vi "Random Strip Chart_v1.vi"() -> ()   [LabVIEW 2026]
panel:
  out "Numeric 3":dbl
  in  "Numeric 2":dbl
  in  "Numeric":dbl
  in  "Loop time (ms)":dbl(knob) scale=0.0..1000.0
  out "Waveform Chart":dbl(graph)
  in  "Stop":bool
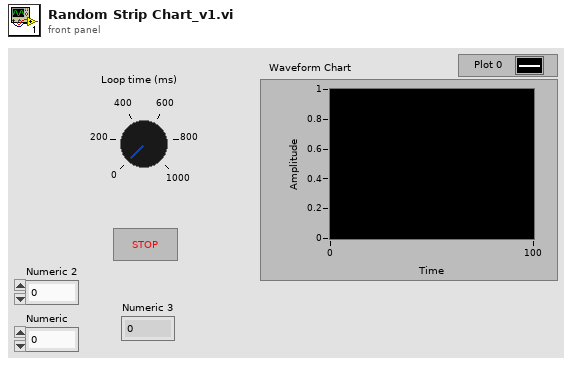
[diagram p1: front panel]
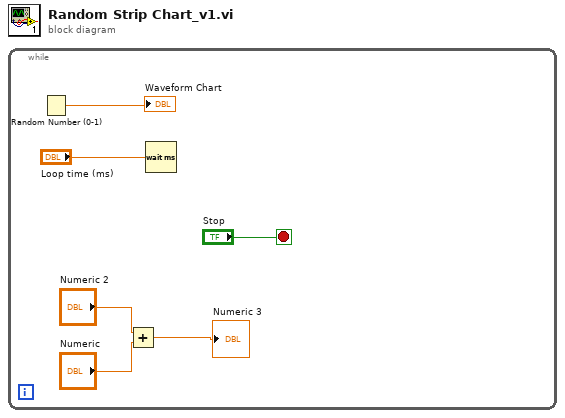
[diagram p0: block diagram]
diagram:
  n1 = while {
    stop <- "Stop" stop-if-true
    n2 = Random Number (0-1)() -> (number: 0 to 1=→"Waveform Chart":dbl)
    n3 = Add(x="Numeric 2", y="Numeric") -> (x+y=→"Numeric 3":dbl)
    n4 = Wait (ms)(milliseconds to wait="Loop time (ms)") -> ()  [unwired: 1 out]
  }
